vi "Query Measurements.vi"() -> ()   [LabVIEW 2024]
uses:
  <vilib>/Plug-In SDKs/Clients/Metadata/Outcome.ctl
  <vilib>/Plug-In SDKs/Clients/Data Store V1/Data Store Client.lvlibp
  <vilib>/Plug-In SDKs/Clients/Metadata/NI Metadata Types.lvlib
panel:
  out "queried measurements":T2(array[cluster])
  in  "odata query":string="$filter=contains(TestResult/Operator/Role, 'Test Engineer')"
  out "error out":errorcluster
  # "Query Measurements\n\nThis example uses the Query Measurements API node with an odata query to display a filtered lists of measurements.\nRun Publish Data.vi to create the data and metadata queried by this VI."
  # "To return all measurements, specify a blank string for odata query."
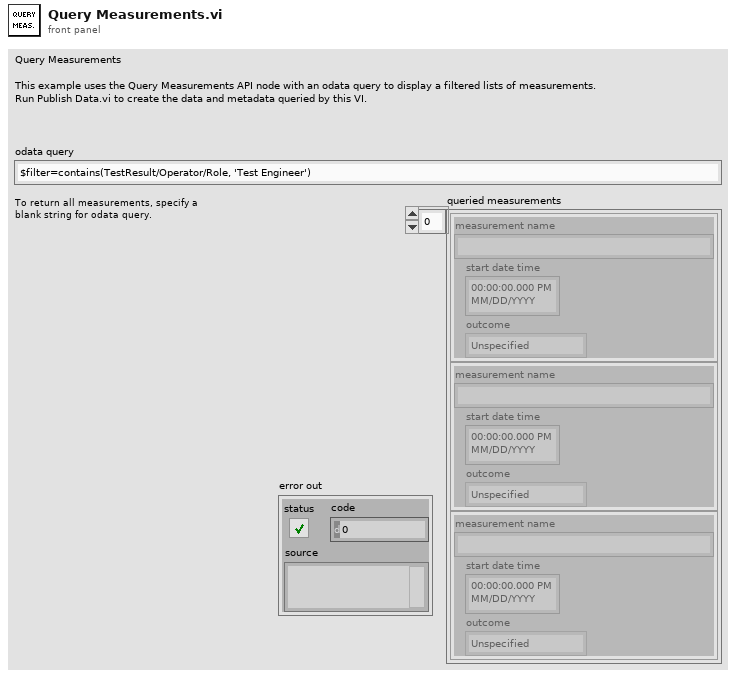
[diagram p1: front panel]
types:
  T1 = typedef "NI Metadata Types.lvlib/Outcome.ctl" = enum32{"Unspecified", "Passed", "Failed", "Indeterminate"}
  T2 = cluster{"measurement name":string, "start date time":timestamp, "outcome":T1}[]
  T3 = typedef "Data Store Client.lvlibp/Published Measurement.ctl" = cluster{"data moniker":T4, "published conditions":T5[], "id":string, "test result id":string, "step id":string, "software item ids":string[], "hardware item ids":string[], "test adapter ids":string[], "name":string, "value type":string, "notes":string, "start date time":timestamp, "end date time":timestamp, "outcome":T1, "parametric index":i32, "error information":T6}
  T4 = typedef "Data Store Client.lvlibp/Data Moniker.ctl" = cluster{"service location":string, "data source":string, "data instance":i64}
  T5 = typedef "Data Store Client.lvlibp/Published Condition.ctl" = cluster{"moniker":T4, "id":string, "name":string, "condition type":string, "step id":string, "test result id":string}
  T6 = typedef "NI Metadata Types.lvlib/Error Information.ctl" = cluster{"error code":i32, "message":string, "source":string}
  T7 = cluster{"name":string, "start date time":timestamp, "outcome":T1}
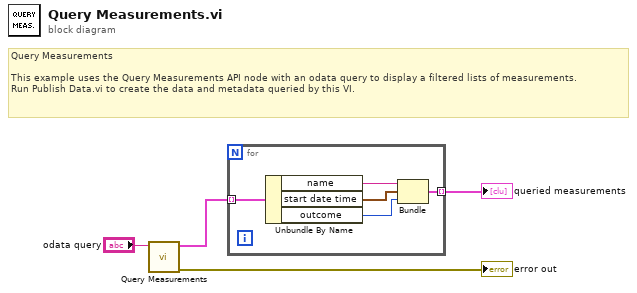
[diagram p0: block diagram]
diagram:
  # "Query Measurements\n\nThis example uses the Query Measurements API node with an odata query to display a filtered lists of measurements.\nRun Publish Data.vi to create the data and metadata queried by this VI."
  n1 = call <vilib>:"Query Measurements.vi"("odata query"="odata query") -> ("error out"=→"error out":errorcluster, "published measurements"=w3:T3[])  [unwired: 9 in]
  n2 = for {
    tunnel: w3 -> [w9] mode=indexing
    tunnel: [w6] -> w2 mode=indexing
    n3 = Unbundle By Name(w9) -> ("name"=w8:string, "start date time"=w7:timestamp, "outcome"=w5:T1)
    n4 = Bundle("name"=w8, "start date time"=w7, "outcome"=w5) -> (w6:T7)  [unwired: 1 in]
  }
  "queried measurements" <- w2
